vi "Set Ref Output.vi"(8 "error in (no error)":errorcluster, 10 "Actual?":T1, 11 "Handle in":i32) -> (0 "error out":errorcluster, 3 "Handle out":i32)   [LabVIEW 2013, in "Thorlabs_MC2000B.lvlib"]
uses:
  <instrlib>/Thorlabs_MC2000B/Thorlabs_MC2000B.lvlib
  <instrlib>/Thorlabs_MC2000B/Public/Advanced/Output mode.ctl
  Program Files/National Instruments/LabVIEW 2011/instr.lib/Thorlabs_MC2000B/Library/MC2000CommandLibWin64.dll
  <instrlib>/Thorlabs_MC2000B/Library/MC2000CommandLibWin32.dll
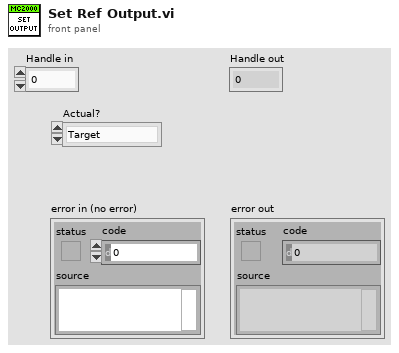
[diagram p1: front panel]
types:
  T1 = typedef "Thorlabs_MC2000B.lvlib/Output mode.ctl" = enum16{"Target", "Actual/Outer", "Inner", "Sum", "Diff"}
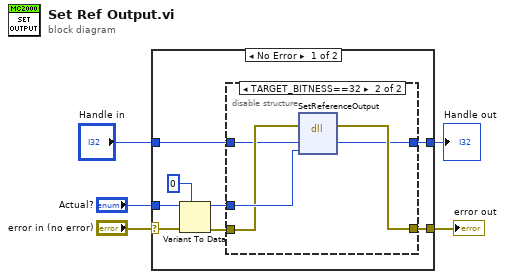
[diagram p0: block diagram]
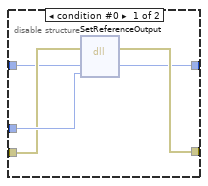
[diagram p2: hidden frame]
diagram:
  n1 = case shown="No Error" "error in (no error)" {
    selector: "error in (no error)" -> [w13 w25]
    tunnel: [w7 w25] -> w5
    tunnel: "Actual?" -> [w12 _]
    tunnel: "Handle in" -> [w8 w24]
    tunnel: [w6 w24] -> w1
    frame No Error {
      n2 = Variant To Data(error in=w13, type=0, Variant=w12) -> (data=w10:i32, error out=w9:errorcluster)
      n3 = disable-structure shown="TARGET_BITNESS==32" {
        disable-tunnel: w10 -> [w18 w23]
        disable-tunnel: w9 -> [w17 w22]
        disable-tunnel: w8 -> [w16 w21]
        disable-tunnel: [w15 w20] -> w7
        disable-tunnel: [w14 w19] -> w6
        frame condition #0 {
          n4 = dll-call lib="D:/Program Files/National Instruments/LabVIEW 2011/instr.lib/Thorlabs_MC2000B/Library/MC2000CommandLibWin64.dll" fn="SetReferenceOutput"(error in=w17, "hdl"=w16, "ref output"=w18) -> (error out=w15:errorcluster, "hdl"=w14:i32)  [unwired: 4 in, 1 out]
        }
        frame condition #1 (active) {
          n5 = dll-call lib="C:/Program Files (x86)/National Instruments/LabVIEW 2013/instr.lib/Thorlabs_MC2000B/Library/MC2000CommandLibWin32.dll" fn="SetReferenceOutput"(error in=w22, "hdl"=w21, "ref output"=w23) -> (error out=w20:errorcluster, "hdl"=w19:i32)  [unwired: 4 in, 1 out]
        }
      }
    }
    frame Error {
    }
  }
  "error out" <- w5
  "Handle out" <- w1
